vi "Driver - DTACQ - Querry Status.vi"(8 "error in":errorcluster, 11 "DTACQ Connection Data In":T3={"Description"="", "Address"="", "Port"=0, "timeout (ms)"=5000, "Termination Character"="\n", "TCP Connection Reference"=refnum, "Open Connection"=FALSE}) -> (0 "error out":errorcluster, 1 "Timed Out":bool=TRUE, 2 "Module Carrier Status":T1, 3 "DTACQ Connection Data Out":T3={"Description"="", "Address"="", "Port"=0, "timeout (ms)"=5000, "Termination Character"="\n", "TCP Connection Reference"=refnum, "Open Connection"=FALSE})   [LabVIEW 2017, in "Communications Library.lvlib"]
doc: "Querries the status from the DTACQ device and interprets the response."
uses:
  Communications Library.lvlib
  Typedefs/DTACQ Connection Data--Cluster.ctl
  Typedefs/DTACQ Module Carrier Status.ctl
  Typedefs/DTACQ Status--Enum.ctl
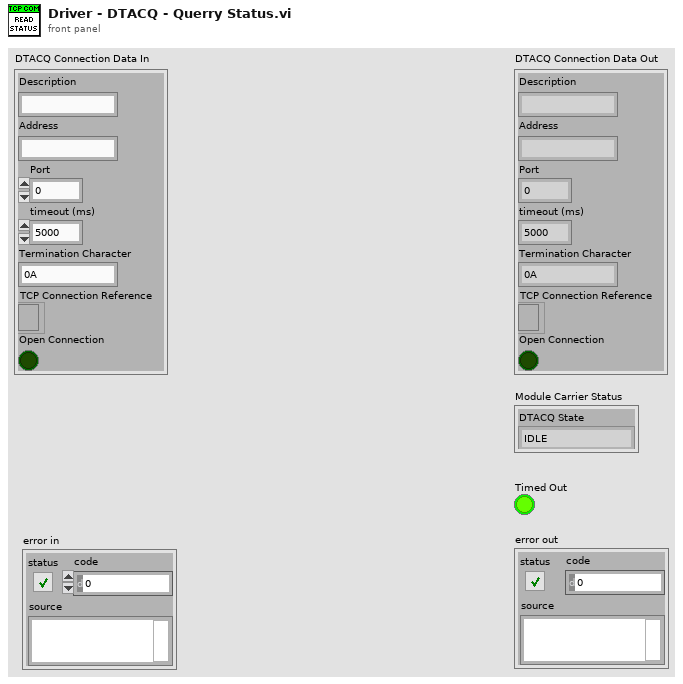
[diagram p1: front panel]
types:
  T1 = typedef "Communications Library.lvlib/DTACQ Module Carrier Status.ctl" = cluster{"DTACQ State":T2, "Pre-Trigger Samples":i32, "Post-Trigger Samples":i32, "Total Samples":i32, "Post Processing":bool}
  T2 = typedef "Communications Library.lvlib/DTACQ Status--Enum.ctl" = enum16{"IDLE", "ARM", "RUN_PRE-TRIGGER", "RUN_POST-TRIGGER", "POST_PROCESS", "CLEANUP"}
  T3 = typedef "Communications Library.lvlib/DTACQ Connection Data--Cluster.ctl" = cluster{"Description":string, "Address":string, "Port":u16, "timeout (ms)":i32, "Termination Character":string, "TCP Connection Reference":refnum<k5>, "Open Connection":bool}
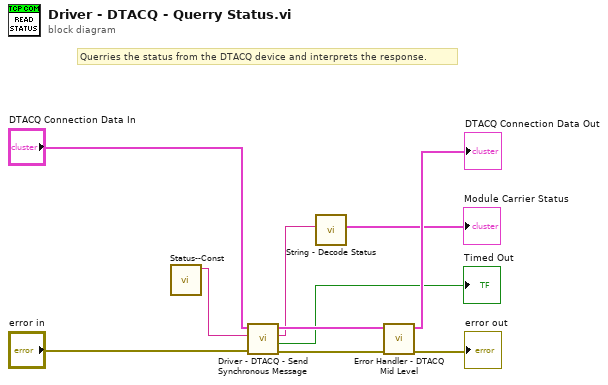
[diagram p0: block diagram]
diagram:
  # "Querries the status from the DTACQ device and interprets the response."
  n1 = call "Status--Const.vi"() -> ("Status Command"=w8:string)  [unwired: 11 in]
  n2 = call "Driver - DTACQ - Send Synchronous Message.vi"("error in"="error in", "Message to Send"=w8, "DTACQ Connection Data In"="DTACQ Connection Data In") -> ("error out"=w6:errorcluster, "Timed Out"=→"Timed Out":bool, "Read String"=w3:string, "DTACQ Connection Data Out"=w4:T3)  [unwired: 5 in]
  n3 = call "String - Decode Status.vi"("Status Response String"=w3) -> ("Module Carrier Status"=→"Module Carrier Status":T1)  [unwired: 9 in, 1 out]
  n4 = call "Error Handler - DTACQ Mid Level.vi"("error in"=w6, "DTACQ Connection Data In"=w4) -> ("error out"=→"error out":errorcluster, "DTACQ Connection Data Out"=→"DTACQ Connection Data Out":T3)  [unwired: 7 in, 1 out]
